vi "Get Timing Info.vi"(8 "error in (no error)":errorcluster, 11 "Channel in":refnum<class "Channel.lvclass">) -> (0 "error out":errorcluster, 1 "Buffer Size":dbl, 2 "Sample Rate":dbl, 3 "Channel out":refnum<class "Channel.lvclass">)   [LabVIEW 2015, in "Channel.lvlib" / "Channel.lvclass"]
uses:
  Channel.lvclass
  ChannelInfo.lvclass
  ChannelConfig.lvclass
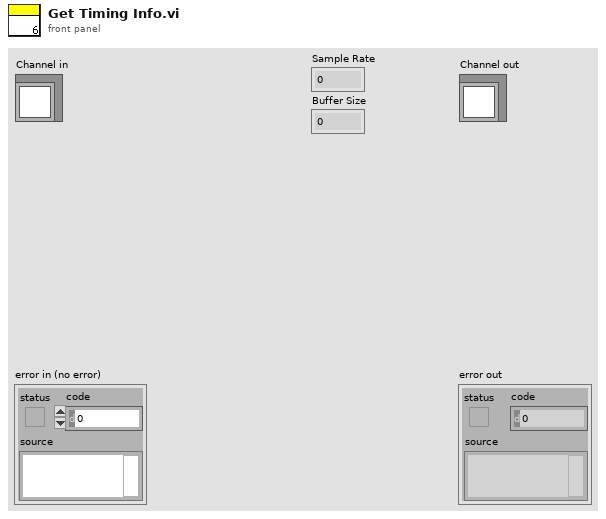
[diagram p1: front panel]
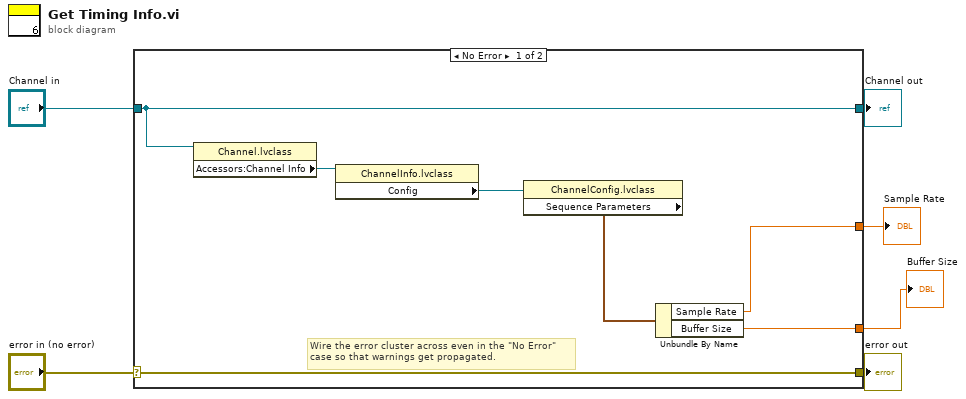
[diagram p0: block diagram]
diagram:
  n1 = case shown="No Error" "error in (no error)" {
    selector: "error in (no error)" -> [w13 w15]
    tunnel: [w13 w15] -> w5
    tunnel: [w10 w14] -> w3
    tunnel: "Channel in" -> [w10 w14]
    tunnel: [w8 _] -> w2
    tunnel: [w7 _] -> w1
    frame No Error {
      # "Wire the error cluster across even in the \"No Error\"\ncase so that warnings get propagated."
      n2 = property class="Channel.lvclass"(reference=w10) -> ("Accessors:Channel Info"=w12:refnum<class "ChannelInfo.lvclass">)  [unwired: 1 in, 2 out]
      n3 = property class="ChannelInfo.lvclass"(reference=w12) -> ("Config"=w11:refnum<class "ChannelConfig.lvclass">)  [unwired: 1 in, 2 out]
      n4 = property class="ChannelConfig.lvclass"(reference=w11) -> ("Sequence Parameters"=w9:cluster{"Buffer Size":dbl, "Sample Rate":dbl})  [unwired: 1 in, 2 out]
      n5 = Unbundle By Name(w9) -> ("Sample Rate"=w8:dbl, "Buffer Size"=w7:dbl)
    }
    frame Error {
    }
  }
  "error out" <- w5
  "Channel out" <- w3
  "Buffer Size" <- w1
  "Sample Rate" <- w2
